vi "CRYImport Calibration Data Dialog.vi"(4 "Invert Curve":bool caption="转化曲线?", 6 "Index":i32, 8 "Calibration In":T1 {"Calibration 2D"."Sens Curve"."Z data" items=["dB", "Lin"]; "Calibration 2D"."Sens Curve"."X data" items=["dB", "Lin"]; "Calibration 2D"."Sens Curve"."Y data" items=["dB", "Lin"]; "Calibration 2D"."Sens Curve"."Z dB ref" format="%.1f"; "Calibration 2D"."Sens Curve"."Z axis" items=["Log", "Lin"]; "Calibration 2D"."Sens Curve"."X dB ref" format="%.1f"; "Calibration 2D"."Sens Curve"."X axis" items=["Log", "Lin"]; "Calibration 2D"."Sens Curve"."Y axis" items=["Log", "Lin"]; "Calibration 2D"."Sens Curve"."Y dB ref" format="%.1f"; "Calibration 2D"."Sens Curve"."Curve"."z" format="%.2f"; "Calibration 2D"."Sens Curve"."Curve"."y" format="%.2f"; "Calibration 2D"."Sens Curve"."Curve"."x" format="%.2f"; "Calibration 2D"."EQ Curve"."Z data" items=["dB", "Lin"]; "Calibration 2D"."EQ Curve"."X data" items=["dB", "Lin"]; "Calibration 2D"."EQ Curve"."Y data" items=["dB", "Lin"]; "Calibration 2D"."EQ Curve"."Z dB ref" format="%.1f"; "Calibration 2D"."EQ Curve"."Z axis" items=["Log", "Lin"]; "Calibration 2D"."EQ Curve"."X dB ref" format="%.1f"; "Calibration 2D"."EQ Curve"."X axis" items=["Log", "Lin"]; "Calibration 2D"."EQ Curve"."Y axis" items=["Log", "Lin"]; "Calibration 2D"."EQ Curve"."Y dB ref" format="%.1f"; "Calibration 2D"."EQ Curve"."Curve"."z" format="%.2f"; "Calibration 2D"."EQ Curve"."Curve"."y" format="%.2f"; "Calibration 2D"."EQ Curve"."Curve"."x" format="%.2f"; "Calibration 2D"."Corr Curve"."Z data" items=["dB", "Lin"]; "Calibration 2D"."Corr Curve"."X data" items=["dB", "Lin"]; "Calibration 2D"."Corr Curve"."Y data" items=["dB", "Lin"]; "Calibration 2D"."Corr Curve"."Z dB ref" format="%.1f"; "Calibration 2D"."Corr Curve"."Z axis" items=["Log", "Lin"]; "Calibration 2D"."Corr Curve"."X dB ref" format="%.1f"; "Calibration 2D"."Corr Curve"."X axis" items=["Log", "Lin"]; "Calibration 2D"."Corr Curve"."Y axis" items=["Log", "Lin"]; "Calibration 2D"."Corr Curve"."Y dB ref" format="%.1f"; "Calibration 2D"."Corr Curve"."Curve"."z" format="%.2f"; "Calibration 2D"."Corr Curve"."Curve"."y" format="%.2f"; "Calibration 2D"."Corr Curve"."Curve"."x" format="%.2f"; "Calibration 2D"."Calibration"."EQ Step size" items=["R10", "R20", "R40", "R80", "User"]; "Calibration 2D"."Calibration"."Corr Step size" items=["R10", "R20", "R40", "R80", "User"]}, 9 "EQ Name":string, 10 "Corr Name":string, 11 "In/Out Channel":bool) -> (0 "Calibration Out":T1 {"Calibration 2D"."Sens Curve"."Z data" items=["dB", "Lin"]; "Calibration 2D"."Sens Curve"."X data" items=["dB", "Lin"]; "Calibration 2D"."Sens Curve"."Y data" items=["dB", "Lin"]; "Calibration 2D"."Sens Curve"."Z dB ref" format="%.1f"; "Calibration 2D"."Sens Curve"."Z axis" items=["Log", "Lin"]; "Calibration 2D"."Sens Curve"."X dB ref" format="%.1f"; "Calibration 2D"."Sens Curve"."X axis" items=["Log", "Lin"]; "Calibration 2D"."Sens Curve"."Y axis" items=["Log", "Lin"]; "Calibration 2D"."Sens Curve"."Y dB ref" format="%.1f"; "Calibration 2D"."Sens Curve"."Curve"."z" format="%.2f"; "Calibration 2D"."Sens Curve"."Curve"."y" format="%.2f"; "Calibration 2D"."Sens Curve"."Curve"."x" format="%.2f"; "Calibration 2D"."EQ Curve"."Z data" items=["dB", "Lin"]; "Calibration 2D"."EQ Curve"."X data" items=["dB", "Lin"]; "Calibration 2D"."EQ Curve"."Y data" items=["dB", "Lin"]; "Calibration 2D"."EQ Curve"."Z dB ref" format="%.1f"; "Calibration 2D"."EQ Curve"."Z axis" items=["Log", "Lin"]; "Calibration 2D"."EQ Curve"."X dB ref" format="%.1f"; "Calibration 2D"."EQ Curve"."X axis" items=["Log", "Lin"]; "Calibration 2D"."EQ Curve"."Y axis" items=["Log", "Lin"]; "Calibration 2D"."EQ Curve"."Y dB ref" format="%.1f"; "Calibration 2D"."EQ Curve"."Curve"."z" format="%.2f"; "Calibration 2D"."EQ Curve"."Curve"."y" format="%.2f"; "Calibration 2D"."EQ Curve"."Curve"."x" format="%.2f"; "Calibration 2D"."Corr Curve"."Z data" items=["dB", "Lin"]; "Calibration 2D"."Corr Curve"."X data" items=["dB", "Lin"]; "Calibration 2D"."Corr Curve"."Y data" items=["dB", "Lin"]; "Calibration 2D"."Corr Curve"."Z dB ref" format="%.1f"; "Calibration 2D"."Corr Curve"."Z axis" items=["Log", "Lin"]; "Calibration 2D"."Corr Curve"."X dB ref" format="%.1f"; "Calibration 2D"."Corr Curve"."X axis" items=["Log", "Lin"]; "Calibration 2D"."Corr Curve"."Y axis" items=["Log", "Lin"]; "Calibration 2D"."Corr Curve"."Y dB ref" format="%.1f"; "Calibration 2D"."Corr Curve"."Curve"."z" format="%.2f"; "Calibration 2D"."Corr Curve"."Curve"."y" format="%.2f"; "Calibration 2D"."Corr Curve"."Curve"."x" format="%.2f"; "Calibration 2D"."Calibration"."EQ Step size" items=["R10", "R20", "R40", "R80", "User"]; "Calibration 2D"."Calibration"."Corr Step size" items=["R10", "R20", "R40", "R80", "User"]}, 3 "Selected Flag":bool)   [LabVIEW 2013]
uses:
  Typedef Control/CRYData Cluster.ctl
  Typedef Control/CRYCalibration All Cluster.ctl
  Typedef Control/CRYCalibration 2DCluster.ctl
  Typedef Control/CRYCalibration Cluster.ctl
panel:
  out "Origin Curve":T4={"Name"="", "Curve"=[], "X data"=1, "Y data"=1, "Z data"=1, "X axis"=0, "Y axis"=1, "Z axis"=1, "X unit"="Hz", "Y unit"="", "Z unit"="deg.", "X dB ref"=1.0, "Y dB ref"=1.0, "Z dB ref"=1.0, "single val"=FALSE, "protected"=FALSE, "display X"=TRUE, "display Y"=TRUE, "display Z"=TRUE, "Test Info"="", "Step No."=0, "Plot Settings"={"Color"=0, "Interpolation"=0, "Point Style"=0, "Line Style"=0, "Point Color"=0, "Line Width"=0, "Bar Plot Style"=0, "Fill To"=0}, "AutoProtect"=FALSE} {"Z data" items=["dB", "Lin"]; "X data" items=["dB", "Lin"]; "Y data" items=["dB", "Lin"]; "Z dB ref" format="%.1f"; "Z axis" items=["Log", "Lin"]; "X dB ref" format="%.1f"; "X axis" items=["Log", "Lin"]; "Y axis" items=["Log", "Lin"]; "Y dB ref" format="%.1f"; "Curve"."z" format="%.2f"; "Curve"."y" format="%.2f"; "Curve"."x" format="%.2f"}
  out "XY Graph":cluster{"XY Graph":cluster{dbl, dbl}[]}[](graph)
  in  "Select Curve Type":enum32{"Equalization", "Correction"}(radio) caption="选择曲线类型"
  in  "Cancel":bool
  in  "OK":bool
  in  "Apply":bool
  out "Destinaton":string caption="目的地"
  in  "Source":u16(ring) caption="原始资料" items=["unity cal-out corr-out", "unity cal-out eq-out", "Crown Amp-L corr-out", "Crown Amp-L eq-out", "Crown Amp-R corr-out", "Crown Amp-R eq-out", "unity cal-in corr-in", "SCM 2 Mic corr-in", "Fundamental"]
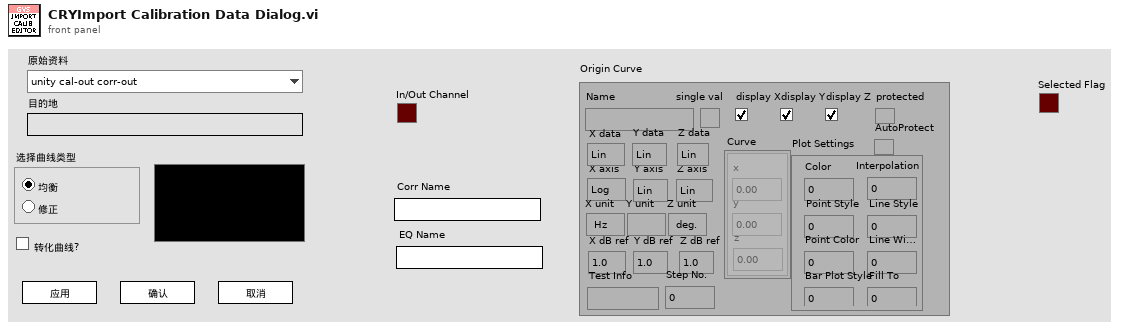
[diagram p1: front panel]
types:
  T1 = typedef "CRYCalibration All Cluster.ctl" = cluster{"Calibration 2D":T2[], "Help":string, "Tab Value":i32, "Input Signal Type":string, "Output Signal Type":string}
  T2 = typedef "CRYCalibration 2DCluster.ctl" = cluster{"Calibration":T3, "Corr Curve":T4, "EQ Curve":T4, "Sens Curve":T4}
  T3 = typedef "CRYCalibration Cluster.ctl" = cluster{"Calibration Step Name":string, "Device":string, "Correction Curve Name":string, "Equalization Curve Name":string, "Sensitivity Curve Name":string, "Corr Folder and File":string, "EQ Folder and File":string, "Sens Folder and File":string, "Corr Step size":u16, "EQ Step size":u16, "Input":bool, "Last Cal Date (sec)":timestamp, "Cha Name":string, "Corr Curve Found":bool, "EQ Curve Found":bool, "Sens Curve Found":bool, "Signal Type":string, "Calibrated Device":string, "Hz":u32}
  T4 = typedef "CRYData Cluster.ctl" = cluster{"Name":string, "Curve":cluster{"x":dbl, "y":dbl, "z":dbl}[], "X data":u16, "Y data":u16, "Z data":u16, "X axis":u16, "Y axis":u16, "Z axis":u16, "X unit":string, "Y unit":string, "Z unit":string, "X dB ref":dbl, "Y dB ref":dbl, "Z dB ref":dbl, "single val":bool, "protected":bool, "display X":bool, "display Y":bool, "display Z":bool, "Test Info":string, "Step No.":i32, "Plot Settings":cluster{"Color":u32, "Interpolation":u8, "Point Style":u8, "Line Style":u8, "Point Color":u32, "Line Width":u8, "Bar Plot Style":u8, "Fill To":i16}, "AutoProtect":bool}
  T5 = enum8{"Enabled", "Disabled", "Disabled and Grayed Out"}
  T6 = typedef "GVSCalibration All Cluster.ctl" = cluster{"Calibration 2D":T7[], "Help":string, "Tab Value":i32, "Input Signal Type":string, "Output Signal Type":string}
  T7 = typedef "GVSCalibration 2DCluster.ctl" = cluster{"Calibration":T8, "Corr Curve":T9, "EQ Curve":T9, "Sens Curve":T9}
  T8 = typedef "GVSCalibration Cluster.ctl" = cluster{"Calibration Step Name":string, "Device":string, "Correction Curve Name":string, "Equalization Curve Name":string, "Sensitivity Curve Name":string, "Corr Folder and File":string, "EQ Folder and File":string, "Sens Folder and File":string, "Corr Step size":u16, "EQ Step size":u16, "Input":bool, "Last Cal Date (sec)":timestamp, "Cha Name":string, "Corr Curve Found":bool, "EQ Curve Found":bool, "Sens Curve Found":bool, "Signal Type":string, "Calibrated Device":string, "Hz":u32}
  T9 = typedef "GVSData Cluster.ctl" = cluster{"Name":string, "Curve":cluster{"x":dbl, "y":dbl, "z":dbl}[], "X data":u16, "Y data":u16, "Z data":u16, "X axis":u16, "Y axis":u16, "Z axis":u16, "X unit":string, "Y unit":string, "Z unit":string, "X dB ref":dbl, "Y dB ref":dbl, "Z dB ref":dbl, "single val":bool, "protected":bool, "display X":bool, "display Y":bool, "display Z":bool, "Test Info":string, "Step No.":i32, "Plot Settings":cluster{"Color":u32, "Interpolation":u8, "Point Style":u8, "Line Style":u8, "Point Color":u32, "Line Width":u8, "Bar Plot Style":u8, "Fill To":i16}, "AutoProtect":bool}
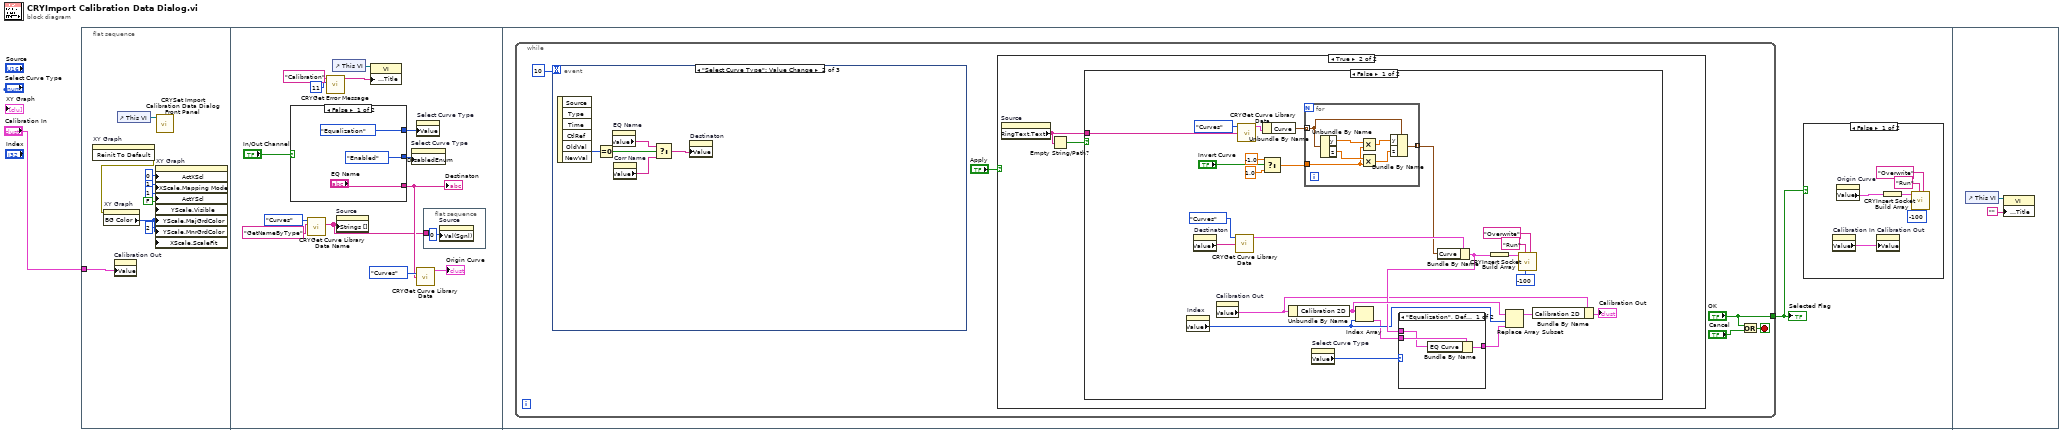
[diagram p0: block diagram]
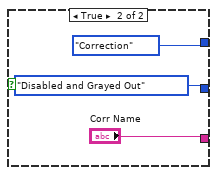
[diagram p2: hidden frame]
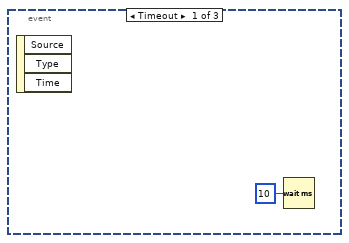
[diagram p4: hidden frame]
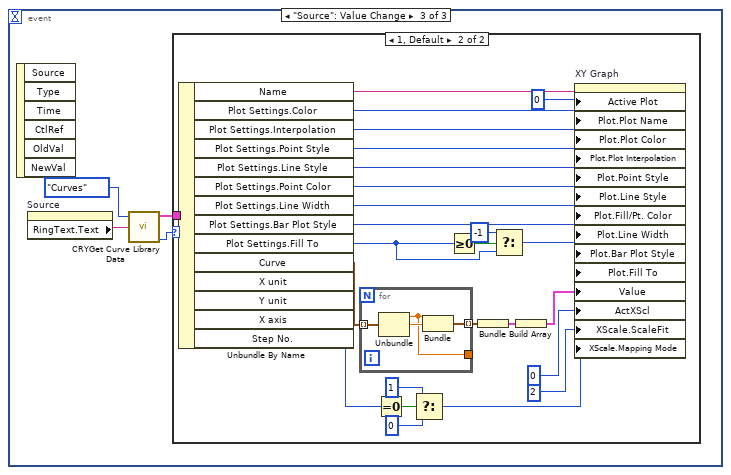
[diagram p5: hidden frame]
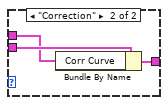
[diagram p8: hidden frame]
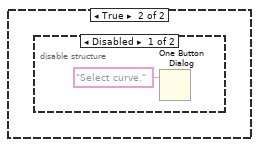
[diagram p9: hidden frame]
diagram:
  n1 = flat-sequence {
    tunnel: "Calibration In" -> [w2]
    frame #0 {
      n2 = invoke on="XY Graph" class="XYGraph (strict)" method="Reinit To Default"() -> (error out=w9:errorcluster)  [unwired: 3 in, 2 out]
      n3 = property on="XY Graph" class="XYGraph (strict)"(error in=w9) -> ("BG Color"=w6:u32)  [unwired: 1 in, 2 out]
      n4 = property on="Calibration Out" class="Clust (strict)"("Value"=w2) -> ()  [unwired: 2 in, 2 out]
      n5 = control-ref of="This VI"() -> (w10:refnum<vi>)
      n6 = property on="XY Graph" class="XYGraph (strict)"("ActXScl"=0 ("Active X Scale"), "XScale.Mapping Mode"=u8 1 ("X Scale.Mapping Mode"), "ActYScl"=1 ("Active Y Scale"), "YScale.Visible"=FALSE ("Y Scale.Visible"), "YScale.MajGrdColor"=w6, "YScale.MnrGrdColor"=w6, "XScale.ScaleFit"=u8 2 ("X Scale.Scale Fit")) -> ()  [unwired: 2 in, 2 out]
      n7 = call "CRYSet Import Calibration Data Dialog Front Panel.vi"("Vi Ref"=w10) -> ()  [unwired: 11 in]
    }
    frame #1 {
      n8 = case shown="False" "In/Out Channel" {
        tunnel: [T5."Enabled" ("Disabled") T5."Disabled and Grayed Out" ("Disabled")] -> w19
        tunnel: [enum32{"Equalization", "Correction"}."Equalization" ("Select Curve Type") enum32{"Equalization", "Correction"}."Correction" ("Select Curve Type")] -> w18
        tunnel: ["EQ Name" "Corr Name"] -> w15
        frame False {
        }
        frame True {
        }
      }
      "Destinaton" <- w15
      n9 = call "CRYGet Curve Library Data Name.vi"("sAction"="GetNameByType", "Type"=enum16{"Curves", "Values", "Results", "WFM"}."Curves") -> ("sNames"=w11:string[])  [unwired: 4 in, 5 out]
      n10 = call "CRYGet Error Message.vi"("Error No"=11, "Kind"="Calibration") -> ("Message"=w12:string)  [unwired: 4 in, 5 out]
      n11 = control-ref of="This VI"() -> (w23:refnum<vi>)
      n12 = property on="Source" class="Ring (strict)"("Strings []"=w11) -> ()  [unwired: 2 in, 2 out]
      n13 = property class="VI"(reference=w23, "Front Panel.Title"=w12) -> ()  [unwired: 1 in, 2 out]
      n14 = property on="Select Curve Type" class="RadioBtnsControl (strict)"("DisabledEnum"=w19) -> ()  [unwired: 2 in, 2 out]
      n15 = property on="Select Curve Type" class="RadioBtnsControl (strict)"("Value"=w18) -> ()  [unwired: 2 in, 2 out]
      n16 = call "CRYGet Curve Library Data.vi"("Type"=enum16{"Curves", "Values", "Results", "WFM"}."Curves", "Data Name"=w15) -> ("Curve"=→"Origin Curve":T4)  [unwired: 4 out]
      n17 = flat-sequence {
        tunnel: w11 -> [_]
        frame #0 {
          n18 = property on="Source" class="Ring (strict)"("Val(Sgnl)"=u16 0 ("Value (Signaling)")) -> ()  [unwired: 2 in, 2 out]
        }
      }
    }
    frame #2 {
      n19 = while {
        tunnel: ["OK"] -> w31
        stop <- w42 stop-if-true
        n20 = event shown="[1] \"Select Curve Type\": Value Change" {
          selector: _ -> [_ _ _]
          dyn-events: _ -> [_ _ _]
          timeout: 10 -> [_ _ _]
          event Timeout {
            n21 = event-data() -> ()  [unwired: 1 in, 3 out]
            n22 = Wait (ms)(milliseconds to wait=u32 10 ("millisecond multiple")) -> ()  [unwired: 1 out]
          }
          event "Select Curve Type": Value Change {
            n23 = event-data() -> ("NewVal"=w48:enum32{"Equalization", "Correction"})  [unwired: 1 in, 5 out]
            n24 = Equal To 0?(x=w48) -> (x = 0?=w47:bool)
            n25 = property on="EQ Name" class="Str"() -> ("Value"=w46:string)  [unwired: 2 in, 2 out]
            n26 = property on="Corr Name" class="Str"() -> ("Value"=w44:string)  [unwired: 2 in, 2 out]
            n27 = Select(t=w46, s=w47, f=w44) -> (s? t:f=w45:string)
            n28 = property on="Destinaton" class="Str"("Value"=w45) -> ()  [unwired: 2 in, 2 out]
          }
          event "Source": Value Change {
            n29 = event-data() -> ()  [unwired: 1 in, 6 out]
            n30 = property on="Source" class="Ring (strict)"() -> ("RingText.Text"=w52:string)  [unwired: 2 in, 2 out]
            n31 = call "CRYGet Curve Library Data.vi"("Type"=enum16{"Curves", "Values", "Results", "WFM"}."Curves", "Data Name"=w52) -> ("Curve"=w50:T4, "index"=w49:i32)  [unwired: 3 out]
            n32 = case shown="1, Default" w49 {
              tunnel: w50 -> [_ w77]
              frame -1 {
              }
              frame 1, Default {
                n33 = Unbundle By Name(w77) -> ("Name"=w75:string, "Plot Settings.Color"=w74:u32, "Plot Settings.Interpolation"=w73:u8, "Plot Settings.Point Style"=w72:u8, "Plot Settings.Line Style"=w71:u8, "Plot Settings.Point Color"=w70:u32, "Plot Settings.Line Width"=w69:u8, "Plot Settings.Bar Plot Style"=w68:u8, "Plot Settings.Fill To"=w54:i16, "Curve"=w65:cluster{"x":dbl, "y":dbl, "z":dbl}[], "X axis"=w58:u16)  [unwired: 3 out]
                n34 = for {
                  tunnel: w65 -> [w80] mode=indexing
                  tunnel: [w79] -> w66 mode=indexing
                  tunnel: [w78] -> _
                  n35 = Unbundle(w80) -> ("x"=w78:dbl, "y"=w81:dbl)  [unwired: 1 out]
                  n36 = Bundle("x"=w78, "y"=w81) -> (w79:cluster{"x":dbl, "y":dbl})  [unwired: 1 out]
                }
                n37 = Equal To 0?(x=w58) -> (x = 0?=w59:bool)
                n38 = Select(t=u8 1, s=w59, f=u8 0) -> (s? t:f=w57:u8)
                n39 = Greater Or Equal To 0?(x=w54) -> (x >= 0?=w55:bool)
                n40 = Bundle(w66) -> (w67:cluster{cluster{"x":dbl, "y":dbl}[]})  [unwired: 1 in]
                n41 = Select(t=i16 -1 ("Fill To"), s=w55, f=w54) -> (s? t:f=w53:i16)
                n42 = Build Array(w67) -> (w64:cluster{cluster{"x":dbl, "y":dbl}[]}[])
                n43 = property on="XY Graph" class="XYGraph (strict)"("Active Plot"=u32 0, "Plot.Plot Name"=w75, "Plot.Plot Color"=w74, "Plot.Plot Interpolation"=w73, "Plot.Point Style"=w72, "Plot.Line Style"=w71, "Plot.Fill/Pt. Color"=w70, "Plot.Line Width"=w69, "Plot.Bar Plot Style"=w68, "Plot.Fill To"=w53, "Value"=w64, "ActXScl"=0 ("Active X Scale"), "XScale.ScaleFit"=u8 2 ("X Scale.Scale Fit"), "XScale.Mapping Mode"=w57) -> ()  [unwired: 2 in, 2 out]
              }
            }
          }
        }
        n44 = case shown="True" "Apply" {
          frame False {
          }
          frame True {
            n45 = property on="Source" class="Ring (strict)"() -> ("RingText.Text"=w82:string)  [unwired: 2 in, 2 out]
            n46 = Empty String/Path?(string/path=w82) -> (empty?=w83:bool)
            n47 = case shown="False" w83 {
              tunnel: w82 -> [w108 _]
              frame False {
                n48 = property on="Index" class="DigNum (strict)"() -> ("Value"=w87:i32)  [unwired: 2 in, 2 out]
                n49 = property on="Destinaton" class="Str"() -> ("Value"=w107:string)  [unwired: 2 in, 2 out]
                n50 = property on="Calibration Out" class="Clust (strict)"() -> ("Value"=w84:T6)  [unwired: 2 in, 2 out]
                n51 = call "CRYGet Curve Library Data.vi"("Type"=enum16{"Curves", "Values", "Results", "WFM"}."Curves", "Data Name"=w107) -> ("Curve"=w106:T4)  [unwired: 4 out]
                n52 = call "CRYGet Curve Library Data.vi"("Type"=enum16{"Curves", "Values", "Results", "WFM"}."Curves", "Data Name"=w108) -> ("Curve"=w98:T4)  [unwired: 4 out]
                n53 = Unbundle By Name(w98) -> ("Curve"=w103:cluster{"x":dbl, "y":dbl, "z":dbl}[])
                n54 = Select(t=-1.0, s="Invert Curve", f=1.0 ("t")) -> (s? t:f=w99:dbl)
                n55 = Unbundle By Name(w84) -> ("Calibration 2D"=w91:T7[])
                n56 = for {
                  tunnel: w103 -> [w121] mode=indexing
                  tunnel: w99 -> [w118]
                  tunnel: [w115] -> w104 mode=indexing
                  n57 = Unbundle By Name(w121) -> ("y"=w120:dbl, "z"=w119:dbl)
                  n58 = Multiply(x=w120, y=w118) -> (x*y=w116:dbl)
                  n59 = Multiply(x=w119, y=w118) -> (x*y=w117:dbl)
                  n60 = Bundle By Name(cluster=w121, "y"=w116, "z"=w117) -> (w115:cluster{"x":dbl, "y":dbl, "z":dbl})
                }
                n61 = property on="Select Curve Type" class="RadioBtnsControl (strict)"() -> ("Value"=w89:enum32{"Equalization", "Correction"})  [unwired: 2 in, 2 out]
                n62 = Index Array(array=w91, index=w87) -> (element=w85:T7)
                n63 = Bundle By Name(cluster=w106, "Curve"=w104) -> (w88:T4)
                n64 = case shown="\"Equalization\", Default" w89 {
                  tunnel: w85 -> [w111 w114]
                  tunnel: [w109 w113] -> w92
                  tunnel: w88 -> [w110 w112]
                  frame "Equalization", Default {
                    n65 = Bundle By Name(cluster=w111, "EQ Curve"=w110) -> (w109:T7)
                  }
                  frame "Correction" {
                    n66 = Bundle By Name(cluster=w114, "Corr Curve"=w112) -> (w113:T7)
                  }
                }
                n67 = Build Array(w88) -> (w94:T4[])
                n68 = Replace Array Subset(array=w91, new element=w92, index=w87) -> (w90:T7[])
                n69 = call "CRYInsert Socket.vi"("sOption2"="Overwrite", "Step No."=-100, "sOption1"="Run" ("sOption"), "Curves"=w94) -> ()  [unwired: 7 in, 1 out]
                n70 = Bundle By Name(cluster=w84, "Calibration 2D"=w90) -> (→"Calibration Out":T6)
              }
              frame True {
                n71 = disable-structure shown="Disabled" {
                  frame Disabled {
                    n72 = One Button Dialog(message="Select curve.") -> ()  [unwired: 1 in, 1 out]
                  }
                  frame Enabled {
                  }
                }
              }
            }
          }
        }
        n73 = Or(x="OK", y="Cancel") -> (x .or. y?=w42:bool)
      }
      "Selected Flag" <- w31
      n74 = case shown="False" w31 {
        frame False {
          n75 = property on="Calibration In" class="Clust (strict)"() -> ("Value"=w32:T6)  [unwired: 2 in, 2 out]
          n76 = property on="Origin Curve" class="Clust (strict)"() -> ("Value"=w37:T9)  [unwired: 2 in, 2 out]
          n77 = property on="Calibration Out" class="Clust (strict)"("Value"=w32) -> ()  [unwired: 2 in, 2 out]
          n78 = Build Array(w37) -> (w34:T9[])
          n79 = call "CRYInsert Socket.vi"("sOption2"="Overwrite", "Step No."=-100, "sOption1"="Run" ("sOption"), "Curves"=w34) -> ()  [unwired: 7 in, 1 out]
        }
        frame True {
        }
      }
    }
    frame #3 {
      n80 = control-ref of="This VI"() -> (w124:refnum<vi>)
      n81 = property class="VI"(reference=w124, "Front Panel.Title"="") -> ()  [unwired: 1 in, 2 out]
    }
  }
